vi "final_control_mk10_040325.vi"() -> ()   [LabVIEW 2023]
doc: "Simplified example program for initializing the COM port, determining the data frame of up to 26 Alicats, acquiring the data of the same number of Alicats, displaying the data of the one with the selected unit ID, and writing a setpoint to the same selected unit ID.\n\nThis is a slightly more feature rich version of the Alicat Simplified Driver Example, and contains an example of a method for interfacing with up to 26 Alicats on a single COM port by means of for loops with shift registers to handle sequential commands to each included Alicat. This also contains a method to write a setpoint to the same selected unit.\n\nIf coding for multiple Alicats on a single COM port without the use of for loops with shift registers, ensure that each Alicat command is executed sequentially. Alicat's RS-232/485 does not work if multiple devices are responding simultaneously."
uses:
  <vilib>/Platform/TimedLoop/XDataNode/timing_clust.ctl
  <vilib>/Platform/TimedLoop/XDataNode/nitl_modes.ctl
  <vilib>/Platform/TimedLoop/XDataNode/wakeup.ctl
  <vilib>/DAQmx/write.llb/DAQmx Write (Analog 1D DBL NChan 1Samp).vi
  <extravilib>/ChannelInstances/Tag-bool/Read With Abort.vi
  <extravilib>/ChannelInstances/Tag-bool/Write With Abort.vi
  <vilib>/Utility/file.llb/Write Delimited Spreadsheet (string).vi
  <extravilib>/ChannelInstances/Tag-bool/Instantiate.vi
  <vilib>/Utility/file.llb/Read Delimited Spreadsheet (DBL).vi
  <extravilib>/ChannelInstances/Tag-bool/EndpointRead.vi
  <vilib>/DAQmx/miscellaneous.llb/DAQmx Fill In Error Info.vi
  <extravilib>/ChannelInstances/Tag-bool/Endpoint.vi
  <vilib>/platform/TimedLoop/XDataNode/XDataNode.xnode
  <vilib>/express/express arith-compare/Formula/XNode/ExpressFormulaBlockNode.xnode
  <vilib>/DAQmx/read.llb/DAQmx Read (Analog DBL 1Chan 1Samp).vi
  <vilib>/Platform/TimedLoop/XDataNode/XDNodeRunTimeDep.lvlib
  <extravilib>/ChannelInstances/Tag-bool.lvlib
panel:
  in  "Tab Control":enum32{"Page 1", "Page 2"}(tab)
  in  "COM Port Settings":T1={"Baud Rate"=enum."19200", "VISA Sesssion In"="MassFlowControllers"}
  out "Range Exceeded":bool
  out "Error Present":bool
  out "Error Text":string
  out "Elapsed Time [ms]\n(all units)":dbl caption="Elapsed Time (s)"
  in  "Minimum time between \nreadings [ms] (all units)":u32
  in  "Device ID's \nto Include:":T2={"A"=TRUE, "B"=TRUE, "C"=TRUE, "D"=TRUE, "E"=TRUE, "F"=TRUE, "G"=FALSE, "H"=FALSE, "I"=FALSE, "J"=FALSE, "K"=FALSE, "L"=FALSE, "M"=FALSE, "N"=FALSE, "O"=FALSE, "P"=FALSE, "Q"=FALSE, "R"=FALSE, "S"=FALSE, "T"=FALSE, "U"=FALSE, "V"=FALSE, "W"=FALSE, "X"=FALSE, "Y"=FALSE, "Z"=FALSE}
  out "Active Device":u16(ring) items=["A", "B", "C", "D", "E", "F"]
  out "Meas. Data (for active device)":T3
  in  "Write File":path
  in  "Hold Time\n[min]":dbl=17.0 min=17.0
  out "N":i32
  in  "Read File":path
  in  "End Program":bool
  in  "Start From:":i32=1
  in  "t_read [ms]":dbl=24000.0
  out "T_SCh [C]":dbl format="%0.2f"
  out "iter start":string
  out "Iter_Duration [ms]":string
  out "C_SP [ppm]":string
  out "C_H2S [ppm]":string
  in  "Start Times":path
  out "len_SP":i32
  out "Setpoints":dbl[][](array[numeric])=[[4.2, 3.3], [69.0, 4.2]]
  out "Z":dbl[](array[numeric])
  out "ASP":dbl
  out "BSP":dbl
  out "CSP":dbl
  out "DSP":dbl
  out "ESP":dbl
  out "FSP":dbl
  out "N_read":i32
  out "Iter_#":string
  out "V_D":string
  out "V_H":string
  out "all rows":dbl[][](array[numeric])
  out "T_SCh":string
  out "Iteration Duration":i64
  out "read_cnt_true":i32
  out "iter_dur_read [ms]":i64
  out "t_diff":dbl
  out "date":string
  out "time":string
  # "Totalizer Timer"
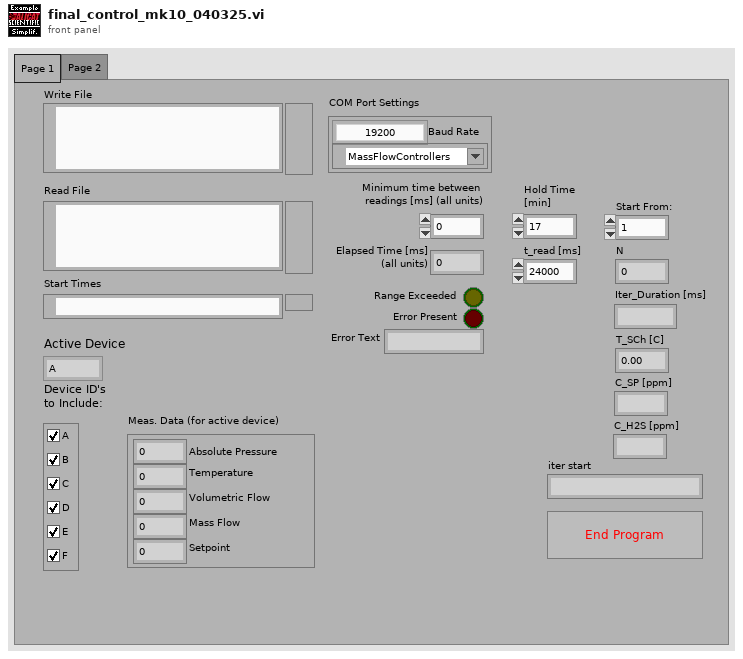
[diagram p1: front panel]
types:
  T1 = cluster{"Baud Rate":enum8{"2400", "9600", "19200", "38400", "57600", "115200", "Unknown"}, "VISA Sesssion In":refnum<visa-resource-name>}
  T2 = cluster{"A":bool, "B":bool, "C":bool, "D":bool, "E":bool, "F":bool, "G":bool, "H":bool, "I":bool, "J":bool, "K":bool, "L":bool, "M":bool, "N":bool, "O":bool, "P":bool, "Q":bool, "R":bool, "S":bool, "T":bool, "U":bool, "V":bool, "W":bool, "X":bool, "Y":bool, "Z":bool}
  T3 = cluster{"Absolute Pressure":dbl, "Gauge/Diff. Pressure":dbl, "Barometric Pressure":dbl, "Temperature":dbl, "Volumetric Flow":dbl, "Mass Flow":dbl, "Setpoint":dbl, "Valve Drive":dbl, "Totalizer":dbl, "[hr]":dbl, "[min]":dbl, "[sec]":dbl, "Totalizer Average Flow":dbl, "Totalizer Peak Flow":dbl, "Gas selected":string}
  T4 = cluster{"Unit ID":string, "Baud Rate":enum8{"2400", "9600", "19200", "38400", "57600", "115200", "Unknown"}, "VISA Sesssion In":refnum<visa-resource-name>}
  T5 = enum16{"Request Ack", "Set Setpoint", "Set Lo Limit", "Set Hi Limit", "Set Prop Band 0-99.9", "Set Integral 0-9.99", "Set Derivative 0-5.0", "Read Int Temp", "Read Ext Temp", "Read Setpoint", "Read Low Limit", "Read High Limit", "Read Prop Band", "Read Integral", "Read Derivative "}
  T6 = typedef "XDNodeRunTimeDep.lvlib/timing_clust.ctl" = cluster{"Expected End [f-1]":u64, "Actual End [f-1]":u64, "Finished Late? [f-1]":bool, "Expected End [i-1]":u64, "Actual End [i-1]":u64, "Finished Late? [i-1]":bool, "Expected Start [i]":u64, "Actual Start [i]":u64, "Expected Start [f]":u64, "Actual Start [f]":u64, "Source Name":string, "Structure Name":string, "Period":i64, "Deadline":i64, "Offset":i64, "Start":i64, "Priority":i32, "Timeout":i32, "Mode":T7, "Wakeup Reason":T8, "Error":errorcluster, "Source Type":string, "Secondary Source Type":string, "Global End Time":u64, "Global Start Time":u64, "Frame Duration":u64, "Iteration Duration":u64, "Assigned CPU":i32, "I/O Scan Engine Mode":u32}
  T7 = typedef "XDNodeRunTimeDep.lvlib/nitl_modes.ctl" = enum32{"No Change", "Process missed periods, maintain original phase", "Discard missed periods, maintain original phase", "Process missed periods, ignore original phase", "Discard missed periods, ignore original phase"}
  T8 = typedef "XDNodeRunTimeDep.lvlib/wakeup.ctl" = enum32{"Normal", "Aborted", "Asynchronous wakeup", "Timing source error", "Timed loop error", "Timeout"}
  T9 = typedef "Tag-bool.lvlib/))Channel.ctl" = refnum<queue>
  T10 = enum8{"2400", "9600", "19200", "38400", "57600", "115200", "Unknown"}
  T11 = cluster{"Absolute Pressure":bool, "Gauge/Diff. Pressure":bool, "Barometric Pressure":bool, "Temperature":bool, "Volumetric":bool, "Mass":bool, "Setpoint":bool, "Valve Drive":bool, "Totalizer":bool, "Totalizer Timer":bool, "Totalizer Average Flow":bool, "Totalizer Peak Flow":bool, "Gas Selected":bool, "Tot. Timer Format":u16}
  T12 = cluster{"Controller Full Scale":dbl, "Controller Select":u16, "Control Range":enum16{"Normal", "Inverted", "Bidirectional", "Unknown"}}
  T13 = cluster{"Controller Full Scale":dbl, "Controller Select":u16, "Control Range":enum16{"Normal", "Inverted", "Bidirectional", "Unknown"}}[]
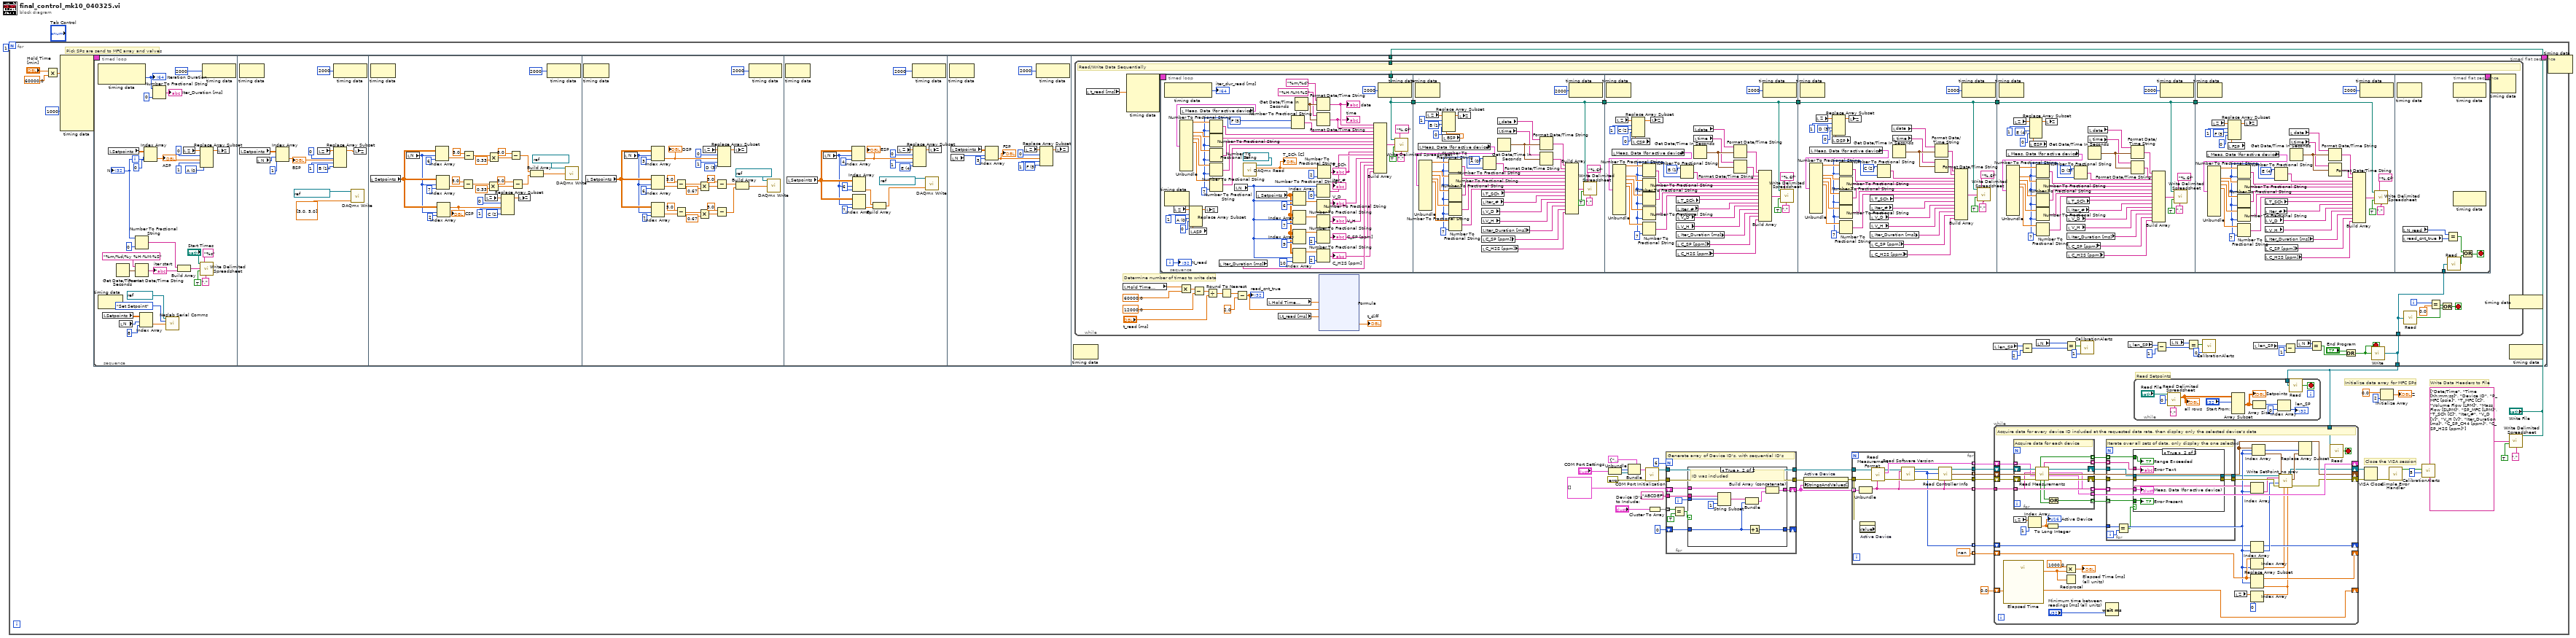
[diagram p0: block diagram]
diagram:
  n1 = for {
    N: 1 -> [_]
    # "Pick SPs are send to MFC array and valves"
    # "Write Data Headers to File"
    # "Read Setpoints"
    # "Initialize data array for MFC SPs"
    # "Close the VISA session"
    n2 = Multiply(x="Hold Time\n[min]", y=60000.0) -> (x*y=w5:dbl)
    n3 = node-c288(w5, i64 1000 ("Offset")) -> (w46:T6)  [unwired: 8 in]
    n4 = timed-loop "Write Data" {
      timing: w46 -> [_]
      timing-out: [_] -> w45
      tunnel: [w59] -> w12
      tunnel: "Write File" -> [w58]
      i -> [w73]
      stop <- w227 stop-if-true
      n5 = timed-sequence {
        timing: _ -> [_]
        timing-out: _ -> [_]
        tunnel: [w61] -> w59
        tunnel: w58 -> [w60]
        n6 = timed-flat-sequence {
          tunnel: [w222] -> w61
          tunnel: w60 -> [w223]
          frame #0 {
            w83 = u16 0 items=["A", "B", "C", "D", "E", "F"]
            n7 = node-c288() -> (w77:i64)  [unwired: 1 in, 1 out]
            "Iteration Duration" <- w77
            n8 = local read "Setpoints"() -> (w67:dbl[][])
            n9 = local read "Setpoints"() -> (w90:dbl[][])
            n10 = Get Date/Time In Seconds() -> (seconds since 1Jan1904=w78:timestamp)
            n11 = local read "N"() -> (w66:i32)
            n12 = Number To Fractional String(number=w73, precision (6)=i16 0) -> (F-format string=w71:string)  [unwired: 2 in]
            n13 = Format Date/Time String(time format string (%c)="%m/%d/%y %H:%M:%S", seconds (now)=w78) -> (date/time string=w70:string)  [unwired: 1 in]
            "iter start" <- w70
            n14 = Index Array(array=w67, index (row)=w66, index (col)=8 ("disabled index (col)")) -> (element=w64:dbl)
            n15 = Index Array(array=w90, index (row)=w73, index (col)=0 ("index (row)")) -> (element=w88:dbl)
            "ASP" <- w88
            n16 = Number To Fractional String(number=w77, precision (6)=i16 0) -> (F-format string=→"Iter_Duration [ms]":string)  [unwired: 2 in]
            n17 = call "Neslab Serial Comms.vi"("VISA resource name"=refnum<visa-resource-name> "COM1", "Command"=T5."Set Setpoint", "Set Value"=w64) -> ()  [unwired: 6 in, 7 out]
            n18 = Build Array(w71, w70) -> (w69:string[])
            n19 = local read "Z"() -> (w86:dbl[])
            n20 = Replace Array Subset(array=w86, new element #1=w88, index #1=0 ("index"), new element #2=w83, index #2=1 ("index")) -> (w87:dbl[])
            n21 = call-poly <vilib>:"Write Delimited Spreadsheet.vi"("file path (dialog if empty)"="Start Times", "format (%s)"="%s" ("format (%.3f)"), "1D data"=w69, "append to file? (new file:F)"=TRUE, "delimiter (\\t)"="," ("delimiter (\\t)")) -> ()  [unwired: 9 in, 2 out]
            n22 = node-c288(i64 2000 ("Start")) -> ()  [unwired: 1 out]
            n23 = local write "Z"(w87) -> ()
            "N" <- w73
          }
          frame #1 {
            w98 = u16 1 items=["A", "B", "C", "D", "E", "F"]
            n24 = node-c288() -> ()  [unwired: 1 in, 1 out]
            n25 = local read "Setpoints"() -> (w106:dbl[][])
            n26 = local read "N"() -> (w99:i32)
            n27 = Index Array(array=w106, index (row)=w99, index (col)=1 ("index (row)")) -> (element=w103:dbl)
            "BSP" <- w103
            n28 = local read "Z"() -> (w101:dbl[])
            n29 = Replace Array Subset(array=w101, new element #1=w103, index #1=0 ("index"), new element #2=w98, index #2=1 ("index")) -> (w102:dbl[])
            n30 = node-c288(i64 2000 ("Start")) -> ()  [unwired: 1 out]
            n31 = call-poly <vilib>:"DAQmx Write.vi"("task/channels in"=refnum<k21> "Valve_cont", "data"=dbl[] [5.0, 5.0]) -> ()  [unwired: 11 in, 3 out]
            n32 = local write "Z"(w102) -> ()
          }
          frame #2 {
            w113 = u16 2 items=["A", "B", "C", "D", "E", "F"]
            n33 = node-c288() -> ()  [unwired: 1 in, 1 out]
            n34 = local read "Setpoints"() -> (w125:dbl[][])
            n35 = local read "N"() -> (w124:i32)
            n36 = Index Array(array=w125, index (row)=w124, index (col)=6 ("disabled index (col)")) -> (element=w115:dbl)
            n37 = Index Array(array=w125, index (row)=w124, index (col)=7 ("disabled index (col)")) -> (element=w123:dbl)
            n38 = Index Array(array=w125, index (row)=w124, index (col)=2 ("index (row)")) -> (element=w137:dbl)
            "CSP" <- w137
            n39 = Subtract(x=5.0, y=w123) -> (x-y=w132:dbl)
            n40 = Subtract(x=5.0, y=w115) -> (x-y=w119:dbl)
            n41 = local read "Z"() -> (w135:dbl[])
            n42 = Multiply(x=w132, y=0.33) -> (x*y=w130:dbl)
            n43 = Multiply(x=w119, y=0.33) -> (x*y=w117:dbl)
            n44 = Replace Array Subset(array=w135, new element #1=w137, index #1=0 ("index"), new element #2=w113, index #2=1 ("index")) -> (w136:dbl[])
            n45 = Subtract(x=5.0, y=w117) -> (x-y=w114:dbl)
            n46 = Subtract(x=5.0, y=w130) -> (x-y=w127:dbl)
            n47 = local write "Z"(w136) -> ()
            n48 = Build Array(w114, w127) -> (w126:dbl[])
            n49 = node-c288(i64 2000 ("Start")) -> ()  [unwired: 1 out]
            n50 = call-poly <vilib>:"DAQmx Write.vi"("task/channels in"=refnum<k21> "Valve_cont", "data"=w126) -> ()  [unwired: 11 in, 3 out]
          }
          frame #3 {
            w164 = u16 3 items=["A", "B", "C", "D", "E", "F"]
            n51 = node-c288() -> ()  [unwired: 1 in, 1 out]
            n52 = local read "Setpoints"() -> (w153:dbl[][])
            n53 = local read "N"() -> (w152:i32)
            n54 = Index Array(array=w153, index (row)=w152, index (col)=7 ("disabled index (col)")) -> (element=w145:dbl)
            n55 = Index Array(array=w153, index (row)=w152, index (col)=3 ("index (row)")) -> (element=w168:dbl)
            "DSP" <- w168
            n56 = Index Array(array=w153, index (row)=w152, index (col)=6 ("disabled index (col)")) -> (element=w151:dbl)
            n57 = Subtract(x=5.0, y=w151) -> (x-y=w161:dbl)
            n58 = Subtract(x=5.0, y=w145) -> (x-y=w149:dbl)
            n59 = Multiply(x=w161, y=0.67) -> (x*y=w159:dbl)
            n60 = Multiply(x=w149, y=0.67) -> (x*y=w147:dbl)
            n61 = local read "Z"() -> (w166:dbl[])
            n62 = Subtract(x=5.0, y=w159) -> (x-y=w155:dbl)
            n63 = Subtract(x=5.0, y=w147) -> (x-y=w144:dbl)
            n64 = Replace Array Subset(array=w166, new element #1=w168, index #1=0 ("index"), new element #2=w164, index #2=1 ("index")) -> (w167:dbl[])
            n65 = local write "Z"(w167) -> ()
            n66 = Build Array(w155, w144) -> (w154:dbl[])
            n67 = node-c288(i64 2000 ("Start")) -> ()  [unwired: 1 out]
            n68 = call-poly <vilib>:"DAQmx Write.vi"("task/channels in"=refnum<k21> "Valve_cont", "data"=w154) -> ()  [unwired: 11 in, 3 out]
          }
          frame #4 {
            w185 = u16 4 items=["A", "B", "C", "D", "E", "F"]
            n69 = node-c288() -> ()  [unwired: 1 in, 1 out]
            n70 = local read "Setpoints"() -> (w180:dbl[][])
            n71 = local read "N"() -> (w179:i32)
            n72 = Index Array(array=w180, index (row)=w179, index (col)=4 ("index (row)")) -> (element=w189:dbl)
            "ESP" <- w189
            n73 = Index Array(array=w180, index (row)=w179, index (col)=6 ("disabled index (col)")) -> (element=w182:dbl)
            n74 = Index Array(array=w180, index (row)=w179, index (col)=7 ("disabled index (col)")) -> (element=w181:dbl)
            n75 = Build Array(w182, w181) -> (w178:dbl[])
            n76 = local read "Z"() -> (w187:dbl[])
            n77 = node-c288(i64 2000 ("Start")) -> ()  [unwired: 1 out]
            n78 = Replace Array Subset(array=w187, new element #1=w189, index #1=0 ("index"), new element #2=w185, index #2=1 ("index")) -> (w188:dbl[])
            n79 = call-poly <vilib>:"DAQmx Write.vi"("task/channels in"=refnum<k21> "Valve_cont", "data"=w178) -> ()  [unwired: 11 in, 3 out]
            n80 = local write "Z"(w188) -> ()
          }
          frame #5 {
            w199 = u16 5 items=["A", "B", "C", "D", "E", "F"]
            n81 = node-c288() -> ()  [unwired: 1 in, 1 out]
            n82 = local read "Setpoints"() -> (w202:dbl[][])
            n83 = local read "N"() -> (w197:i32)
            n84 = Index Array(array=w202, index (row)=w197, index (col)=5 ("index (row)")) -> (element=w198:dbl)
            "FSP" <- w198
            n85 = local read "Z"() -> (w201:dbl[])
            n86 = node-c288(i64 2000 ("Start")) -> ()  [unwired: 1 out]
            n87 = Replace Array Subset(array=w201, new element #1=w198, index #1=0 ("index"), new element #2=w199, index #2=1 ("index")) -> (w200:dbl[])
            n88 = local write "Z"(w200) -> ()
          }
          frame #6 {
            n89 = node-c288() -> ()  [unwired: 1 in, 1 out]
            n90 = local read "len_SP"() -> (w213:i32)
            n91 = Subtract(x=w213, y=2) -> (x-y=w215:i32)
            n92 = local read "N"() -> (w214:i32)
            n93 = Equal?(x=w214, y=w215) -> (x = y?=w211:bool)
            n94 = call "CalibrationAlerts.vi"("Alert Type (0)"=1, "Trigger"=w211) -> ()  [unwired: 10 in]
            n95 = local read "len_SP"() -> (w218:i32)
            n96 = Subtract(x=w218, y=1) -> (x-y=w217:i32)
            n97 = local read "N"() -> (w221:i32)
            n98 = Equal?(x=w221, y=w217) -> (x = y?=w210:bool)
            n99 = call "CalibrationAlerts.vi"("Alert Type (0)"=0, "Trigger"=w210) -> ()  [unwired: 10 in]
            n100 = local read "len_SP"() -> (w226:i32)
            n101 = Subtract(x=w226, y=1) -> (x-y=w229:i32)
            n102 = local read "N"() -> (w225:i32)
            n103 = Equal?(x=w225, y=w229) -> (x = y?=w228:bool)
            n104 = Or(x="End Program", y=w228) -> (x .or. y?=w227:bool)
            n105 = call <extravilib>:"Write.vi"("element"=w227) -> ("channel"=w222:T9)  [unwired: 1 out]
            n106 = while {
              tunnel: w223 -> [w251]
              tunnel: w222 -> [w241]
              i -> [w240]
              stop <- w247 stop-if-true
              # "Determine number of times to write data"
              # "Read/Write Data Sequentially"
              n107 = local read "t_read [ms]"() -> (w231:dbl)
              n108 = local read "Hold Time\n[min]"() -> (w245:dbl)
              n109 = node-c288(w231) -> (w253:T6)  [unwired: 3 in]
              n110 = timed-loop {
                timing: w253 -> [_]
                timing-out: [_] -> w252
                tunnel: w251 -> [w266]
                tunnel: w241 -> [w267]
                i -> [w330]
                stop <- w549 stop-if-true
                n111 = timed-sequence {
                  timing: _ -> [_]
                  timing-out: _ -> [_]
                  tunnel: w267 -> [w269]
                  tunnel: w266 -> [w268]
                  n112 = timed-flat-sequence {
                    tunnel: [w296] -> w274
                    tunnel: w268 -> [w296]
                    tunnel: w274 -> [w361]
                    tunnel: [w361] -> w273
                    tunnel: w273 -> [w396]
                    tunnel: [w396] -> w272
                    tunnel: w272 -> [w434]
                    tunnel: [w434] -> w271
                    tunnel: w271 -> [w466]
                    tunnel: [w466] -> w270
                    tunnel: w270 -> [w518]
                    tunnel: w269 -> [w548]
                    frame #0 {
                      w311 = u16 5 items=["A", "B", "C", "D", "E", "F"]
                      w314 = u16 0 items=["A", "B", "C", "D", "E", "F"]
                      w307 = i16 7 ("precision (6)")
                      n113 = node-c288() -> (→"iter_dur_read [ms]":i64)  [unwired: 1 in]
                      n114 = local read "Z"() -> (w300:dbl[])
                      n115 = local read "Meas. Data (for active device)"() -> (w297:T3)
                      n116 = Unbundle(w297) -> ("Absolute Pressure"=w320:dbl, "Temperature"=w310:dbl, "Volumetric Flow"=w316:dbl, "Mass Flow"=w309:dbl, "Setpoint"=w308:dbl)  [unwired: 10 out]
                      n117 = local read "ASP"() -> (w298:dbl)
                      n118 = Replace Array Subset(array=w300, new element #1=w314, index #1=1 ("index"), new element #2=w298, index #2=0 ("index")) -> (w299:dbl[])
                      n119 = local write "Z"(w299) -> ()
                      n120 = Number To Fractional String(number=w320, precision (6)=w307) -> (F-format string=w305:string)  [unwired: 2 in]
                      n121 = Number To Fractional String(number=w310, precision (6)=w307) -> (F-format string=w303:string)  [unwired: 2 in]
                      n122 = Number To Fractional String(number=w316, precision (6)=w307) -> (F-format string=w304:string)  [unwired: 2 in]
                      n123 = Number To Fractional String(number=w309, precision (6)=w307) -> (F-format string=w302:string)  [unwired: 2 in]
                      n124 = Number To Fractional String(number=w308, precision (6)=w307) -> (F-format string=w301:string)  [unwired: 2 in]
                      n125 = local read "Iter_Duration [ms]"() -> (w295:string)
                      n126 = local read "N"() -> (w277:i32)
                      n127 = call-poly <vilib>:"DAQmx Read.vi"("task/channels in"=refnum<k21> "T_SCh") -> ("data"=w323:dbl)  [unwired: 12 in, 2 out]
                      "T_SCh [C]" <- w323
                      n128 = local read "Setpoints"() -> (w276:dbl[][])
                      n129 = Number To Fractional String(number=w311, precision (6)=w307) -> (F-format string=w306:string)  [unwired: 2 in]
                      n130 = Index Array(array=w276, index (row)=w277, index (col)=6 ("disabled index (col)")) -> (element=w327:dbl)
                      n131 = Index Array(array=w276, index (row)=w277, index (col)=7 ("disabled index (col)")) -> (element=w326:dbl)
                      n132 = Index Array(array=w276, index (row)=w277, index (col)=9 ("disabled index (col)")) -> (element=w283:dbl)
                      n133 = Index Array(array=w276, index (row)=w277, index (col)=10 ("disabled index (col)")) -> (element=w279:dbl)
                      n134 = Get Date/Time In Seconds() -> (seconds since 1Jan1904=w289:timestamp)
                      n135 = Format Date/Time String(time format string (%c)="%m/%d", seconds (now)=w289) -> (date/time string=w291:string)  [unwired: 1 in]
                      "date" <- w291
                      n136 = Format Date/Time String(time format string (%c)="%H:%M:%S", seconds (now)=w289) -> (date/time string=w290:string)  [unwired: 1 in]
                      "time" <- w290
                      n137 = Number To Fractional String(number=w277, precision (6)=i16 0) -> (F-format string=w292:string)  [unwired: 2 in]
                      "Iter_#" <- w292
                      n138 = Number To Fractional String(number=w327) -> (F-format string=w293:string)  [unwired: 3 in]
                      "V_D" <- w293
                      n139 = Number To Fractional String(number=w326) -> (F-format string=w294:string)  [unwired: 3 in]
                      "V_H" <- w294
                      n140 = Number To Fractional String(number=w283, precision (6)=i16 2) -> (F-format string=w281:string)  [unwired: 2 in]
                      "C_SP [ppm]" <- w281
                      n141 = Number To Fractional String(number=w279, precision (6)=i16 2) -> (F-format string=w275:string)  [unwired: 2 in]
                      "C_H2S [ppm]" <- w275
                      n142 = Number To Fractional String(number=w323, precision (6)=i16 2) -> (F-format string=w286:string)  [unwired: 2 in]
                      "T_SCh" <- w286
                      n143 = Build Array(w291, w290, w306, w305, w303, w304, w302, w301, w286, w292, w293, w294, w295, w281, w275) -> (w317:string[])
                      n144 = node-c288(i64 2000 ("Start")) -> ()  [unwired: 1 out]
                      n145 = call-poly <vilib>:"Write Delimited Spreadsheet.vi"("file path (dialog if empty)"=w296, "format (%s)"="%.6f" ("format (%.3f)"), "1D data"=w317, "append to file? (new file:F)"=TRUE, "delimiter (\\t)"="," ("delimiter (\\t)")) -> ()  [unwired: 9 in, 2 out]
                      "N_read" <- w330
                    }
                    frame #1 {
                      w358 = u16 0 items=["A", "B", "C", "D", "E", "F"]
                      w367 = u16 1 items=["A", "B", "C", "D", "E", "F"]
                      w354 = i16 7 ("precision (6)")
                      n146 = node-c288() -> ()  [unwired: 1 in, 1 out]
                      n147 = local read "Meas. Data (for active device)"() -> (w365:T3)
                      n148 = Unbundle(w365) -> ("Absolute Pressure"=w373:dbl, "Temperature"=w357:dbl, "Volumetric Flow"=w369:dbl, "Mass Flow"=w356:dbl, "Setpoint"=w355:dbl)  [unwired: 10 out]
                      n149 = local read "Z"() -> (w364:dbl[])
                      n150 = local read "BSP"() -> (w359:dbl)
                      n151 = Replace Array Subset(array=w364, new element #1=w367, index #1=1 ("index"), new element #2=w359, index #2=0 ("index")) -> (w363:dbl[])
                      n152 = Number To Fractional String(number=w373, precision (6)=w354) -> (F-format string=w352:string)  [unwired: 2 in]
                      n153 = Number To Fractional String(number=w357, precision (6)=w354) -> (F-format string=w350:string)  [unwired: 2 in]
                      n154 = Number To Fractional String(number=w369, precision (6)=w354) -> (F-format string=w351:string)  [unwired: 2 in]
                      n155 = Number To Fractional String(number=w356, precision (6)=w354) -> (F-format string=w349:string)  [unwired: 2 in]
                      n156 = Number To Fractional String(number=w355, precision (6)=w354) -> (F-format string=w348:string)  [unwired: 2 in]
                      n157 = local write "Z"(w363) -> ()
                      n158 = local read "T_SCh"() -> (w347:string)
                      n159 = local read "Iter_#"() -> (w346:string)
                      n160 = local read "V_D"() -> (w345:string)
                      n161 = local read "V_H"() -> (w344:string)
                      n162 = local read "Iter_Duration [ms]"() -> (w343:string)
                      n163 = local read "C_SP [ppm]"() -> (w337:string)
                      n164 = local read "C_H2S [ppm]"() -> (w336:string)
                      n165 = Number To Fractional String(number=w358, precision (6)=w354) -> (F-format string=w353:string)  [unwired: 2 in]
                      n166 = local read "date"() -> (w338:string)
                      n167 = local read "time"() -> (w339:string)
                      n168 = Get Date/Time In Seconds() -> (seconds since 1Jan1904=w340:timestamp)
                      n169 = Format Date/Time String(time format string (%c)=w338, seconds (now)=w340) -> (date/time string=w342:string)  [unwired: 1 in]
                      n170 = Format Date/Time String(time format string (%c)=w339, seconds (now)=w340) -> (date/time string=w341:string)  [unwired: 1 in]
                      n171 = Build Array(w342, w341, w353, w352, w350, w351, w349, w348, w347, w346, w345, w344, w343, w337, w336) -> (w370:string[])
                      n172 = node-c288(i64 2000 ("Start")) -> ()  [unwired: 1 out]
                      n173 = call-poly <vilib>:"Write Delimited Spreadsheet.vi"("file path (dialog if empty)"=w361, "format (%s)"="%.6f" ("format (%.3f)"), "1D data"=w370, "append to file? (new file:F)"=TRUE, "delimiter (\\t)"="," ("delimiter (\\t)")) -> ()  [unwired: 9 in, 2 out]
                    }
                    frame #2 {
                      w402 = u16 1 items=["A", "B", "C", "D", "E", "F"]
                      w401 = i16 7 ("precision (6)")
                      w414 = u16 2 items=["A", "B", "C", "D", "E", "F"]
                      n174 = node-c288() -> ()  [unwired: 1 in, 1 out]
                      n175 = local read "Meas. Data (for active device)"() -> (w403:T3)
                      n176 = Unbundle(w403) -> ("Absolute Pressure"=w408:dbl, "Temperature"=w406:dbl, "Volumetric Flow"=w407:dbl, "Mass Flow"=w405:dbl, "Setpoint"=w404:dbl)  [unwired: 10 out]
                      n177 = local read "Z"() -> (w413:dbl[])
                      n178 = local read "CSP"() -> (w409:dbl)
                      n179 = Replace Array Subset(array=w413, new element #1=w414, index #1=1 ("index"), new element #2=w409, index #2=0 ("index")) -> (w412:dbl[])
                      n180 = Number To Fractional String(number=w408, precision (6)=w401) -> (F-format string=w389:string)  [unwired: 2 in]
                      n181 = Number To Fractional String(number=w406, precision (6)=w401) -> (F-format string=w388:string)  [unwired: 2 in]
                      n182 = Number To Fractional String(number=w407, precision (6)=w401) -> (F-format string=w387:string)  [unwired: 2 in]
                      n183 = Number To Fractional String(number=w405, precision (6)=w401) -> (F-format string=w386:string)  [unwired: 2 in]
                      n184 = Number To Fractional String(number=w404, precision (6)=w401) -> (F-format string=w385:string)  [unwired: 2 in]
                      n185 = local write "Z"(w412) -> ()
                      n186 = local read "T_SCh"() -> (w395:string)
                      n187 = local read "Iter_#"() -> (w394:string)
                      n188 = local read "V_D"() -> (w393:string)
                      n189 = local read "V_H"() -> (w392:string)
                      n190 = local read "Iter_Duration [ms]"() -> (w391:string)
                      n191 = local read "C_SP [ppm]"() -> (w379:string)
                      n192 = local read "C_H2S [ppm]"() -> (w378:string)
                      n193 = Number To Fractional String(number=w402, precision (6)=w401) -> (F-format string=w390:string)  [unwired: 2 in]
                      n194 = local read "date"() -> (w380:string)
                      n195 = local read "time"() -> (w381:string)
                      n196 = Get Date/Time In Seconds() -> (seconds since 1Jan1904=w382:timestamp)
                      n197 = Format Date/Time String(time format string (%c)=w380, seconds (now)=w382) -> (date/time string=w384:string)  [unwired: 1 in]
                      n198 = Format Date/Time String(time format string (%c)=w381, seconds (now)=w382) -> (date/time string=w383:string)  [unwired: 1 in]
                      n199 = Build Array(w384, w383, w390, w389, w388, w387, w386, w385, w395, w394, w393, w392, w391, w379, w378) -> (w397:string[])
                      n200 = node-c288(i64 2000 ("Start")) -> ()  [unwired: 1 out]
                      n201 = call-poly <vilib>:"Write Delimited Spreadsheet.vi"("file path (dialog if empty)"=w396, "format (%s)"="%.6f" ("format (%.3f)"), "1D data"=w397, "append to file? (new file:F)"=TRUE, "delimiter (\\t)"="," ("delimiter (\\t)")) -> ()  [unwired: 9 in, 2 out]
                    }
                    frame #3 {
                      w428 = u16 3 items=["A", "B", "C", "D", "E", "F"]
                      w451 = u16 2 items=["A", "B", "C", "D", "E", "F"]
                      w450 = i16 7 ("precision (6)")
                      n202 = node-c288() -> ()  [unwired: 1 in, 1 out]
                      n203 = local read "Meas. Data (for active device)"() -> (w433:T3)
                      n204 = Unbundle(w433) -> ("Absolute Pressure"=w456:dbl, "Temperature"=w454:dbl, "Volumetric Flow"=w455:dbl, "Mass Flow"=w453:dbl, "Setpoint"=w452:dbl)  [unwired: 10 out]
                      n205 = local read "Z"() -> (w431:dbl[])
                      n206 = local read "DSP"() -> (w432:dbl)
                      n207 = Replace Array Subset(array=w431, new element #1=w428, index #1=1 ("index"), new element #2=w432, index #2=0 ("index")) -> (w430:dbl[])
                      n208 = Number To Fractional String(number=w456, precision (6)=w450) -> (F-format string=w444:string)  [unwired: 2 in]
                      n209 = Number To Fractional String(number=w454, precision (6)=w450) -> (F-format string=w443:string)  [unwired: 2 in]
                      n210 = Number To Fractional String(number=w455, precision (6)=w450) -> (F-format string=w442:string)  [unwired: 2 in]
                      n211 = Number To Fractional String(number=w453, precision (6)=w450) -> (F-format string=w441:string)  [unwired: 2 in]
                      n212 = Number To Fractional String(number=w452, precision (6)=w450) -> (F-format string=w440:string)  [unwired: 2 in]
                      n213 = local write "Z"(w430) -> ()
                      n214 = local read "T_SCh"() -> (w435:string)
                      n215 = local read "Iter_#"() -> (w436:string)
                      n216 = local read "V_D"() -> (w437:string)
                      n217 = local read "V_H"() -> (w438:string)
                      n218 = local read "Iter_Duration [ms]"() -> (w439:string)
                      n219 = local read "C_SP [ppm]"() -> (w421:string)
                      n220 = local read "C_H2S [ppm]"() -> (w420:string)
                      n221 = Number To Fractional String(number=w451, precision (6)=w450) -> (F-format string=w445:string)  [unwired: 2 in]
                      n222 = local read "date"() -> (w422:string)
                      n223 = local read "time"() -> (w423:string)
                      n224 = Get Date/Time In Seconds() -> (seconds since 1Jan1904=w424:timestamp)
                      n225 = Format Date/Time String(time format string (%c)=w422, seconds (now)=w424) -> (date/time string=w426:string)  [unwired: 1 in]
                      n226 = Format Date/Time String(time format string (%c)=w423, seconds (now)=w424) -> (date/time string=w425:string)  [unwired: 1 in]
                      n227 = Build Array(w426, w425, w445, w444, w443, w442, w441, w440, w435, w436, w437, w438, w439, w421, w420) -> (w446:string[])
                      n228 = node-c288(i64 2000 ("Start")) -> ()  [unwired: 1 out]
                      n229 = call-poly <vilib>:"Write Delimited Spreadsheet.vi"("file path (dialog if empty)"=w434, "format (%s)"="%.6f" ("format (%.3f)"), "1D data"=w446, "append to file? (new file:F)"=TRUE, "delimiter (\\t)"="," ("delimiter (\\t)")) -> ()  [unwired: 9 in, 2 out]
                    }
                    frame #4 {
                      w474 = u16 4 items=["A", "B", "C", "D", "E", "F"]
                      w493 = u16 3 items=["A", "B", "C", "D", "E", "F"]
                      w492 = i16 7 ("precision (6)")
                      n230 = node-c288() -> ()  [unwired: 1 in, 1 out]
                      n231 = local read "Meas. Data (for active device)"() -> (w476:T3)
                      n232 = Unbundle(w476) -> ("Absolute Pressure"=w498:dbl, "Temperature"=w496:dbl, "Volumetric Flow"=w497:dbl, "Mass Flow"=w495:dbl, "Setpoint"=w494:dbl)  [unwired: 10 out]
                      n233 = local read "Z"() -> (w471:dbl[])
                      n234 = local read "ESP"() -> (w472:dbl)
                      n235 = Replace Array Subset(array=w471, new element #1=w474, index #1=1 ("index"), new element #2=w472, index #2=0 ("index")) -> (w470:dbl[])
                      n236 = Number To Fractional String(number=w498, precision (6)=w492) -> (F-format string=w486:string)  [unwired: 2 in]
                      n237 = Number To Fractional String(number=w496, precision (6)=w492) -> (F-format string=w485:string)  [unwired: 2 in]
                      n238 = Number To Fractional String(number=w497, precision (6)=w492) -> (F-format string=w484:string)  [unwired: 2 in]
                      n239 = Number To Fractional String(number=w495, precision (6)=w492) -> (F-format string=w483:string)  [unwired: 2 in]
                      n240 = Number To Fractional String(number=w494, precision (6)=w492) -> (F-format string=w482:string)  [unwired: 2 in]
                      n241 = local write "Z"(w470) -> ()
                      n242 = local read "T_SCh"() -> (w481:string)
                      n243 = local read "Iter_#"() -> (w477:string)
                      n244 = local read "V_D"() -> (w478:string)
                      n245 = local read "V_H"() -> (w479:string)
                      n246 = local read "Iter_Duration [ms]"() -> (w480:string)
                      n247 = local read "C_SP [ppm]"() -> (w463:string)
                      n248 = local read "C_H2S [ppm]"() -> (w462:string)
                      n249 = Number To Fractional String(number=w493, precision (6)=w492) -> (F-format string=w487:string)  [unwired: 2 in]
                      n250 = local read "date"() -> (w464:string)
                      n251 = local read "time"() -> (w465:string)
                      n252 = Get Date/Time In Seconds() -> (seconds since 1Jan1904=w467:timestamp)
                      n253 = Format Date/Time String(time format string (%c)=w464, seconds (now)=w467) -> (date/time string=w469:string)  [unwired: 1 in]
                      n254 = Format Date/Time String(time format string (%c)=w465, seconds (now)=w467) -> (date/time string=w468:string)  [unwired: 1 in]
                      n255 = Build Array(w469, w468, w487, w486, w485, w484, w483, w482, w481, w477, w478, w479, w480, w463, w462) -> (w488:string[])
                      n256 = node-c288(i64 2000 ("Start")) -> ()  [unwired: 1 out]
                      n257 = call-poly <vilib>:"Write Delimited Spreadsheet.vi"("file path (dialog if empty)"=w466, "format (%s)"="%.6f" ("format (%.3f)"), "1D data"=w488, "append to file? (new file:F)"=TRUE, "delimiter (\\t)"="," ("delimiter (\\t)")) -> ()  [unwired: 9 in, 2 out]
                    }
                    frame #5 {
                      w516 = u16 5 items=["A", "B", "C", "D", "E", "F"]
                      w536 = u16 4 items=["A", "B", "C", "D", "E", "F"]
                      w535 = i16 7 ("precision (6)")
                      n258 = node-c288() -> ()  [unwired: 1 in, 1 out]
                      n259 = local read "Meas. Data (for active device)"() -> (w519:T3)
                      n260 = Unbundle(w519) -> ("Absolute Pressure"=w541:dbl, "Temperature"=w539:dbl, "Volumetric Flow"=w540:dbl, "Mass Flow"=w538:dbl, "Setpoint"=w537:dbl)  [unwired: 10 out]
                      n261 = local read "Z"() -> (w512:dbl[])
                      n262 = local read "FSP"() -> (w514:dbl)
                      n263 = Replace Array Subset(array=w512, new element #1=w516, index #1=1 ("index"), new element #2=w514, index #2=0 ("index")) -> (w513:dbl[])
                      n264 = Number To Fractional String(number=w541, precision (6)=w535) -> (F-format string=w529:string)  [unwired: 2 in]
                      n265 = Number To Fractional String(number=w539, precision (6)=w535) -> (F-format string=w528:string)  [unwired: 2 in]
                      n266 = Number To Fractional String(number=w540, precision (6)=w535) -> (F-format string=w527:string)  [unwired: 2 in]
                      n267 = Number To Fractional String(number=w538, precision (6)=w535) -> (F-format string=w526:string)  [unwired: 2 in]
                      n268 = Number To Fractional String(number=w537, precision (6)=w535) -> (F-format string=w525:string)  [unwired: 2 in]
                      n269 = local write "Z"(w513) -> ()
                      n270 = local read "T_SCh"() -> (w520:string)
                      n271 = local read "Iter_#"() -> (w521:string)
                      n272 = local read "V_D"() -> (w522:string)
                      n273 = local read "V_H"() -> (w523:string)
                      n274 = local read "Iter_Duration [ms]"() -> (w524:string)
                      n275 = local read "C_SP [ppm]"() -> (w506:string)
                      n276 = local read "C_H2S [ppm]"() -> (w505:string)
                      n277 = Number To Fractional String(number=w536, precision (6)=w535) -> (F-format string=w530:string)  [unwired: 2 in]
                      n278 = local read "date"() -> (w507:string)
                      n279 = local read "time"() -> (w508:string)
                      n280 = Get Date/Time In Seconds() -> (seconds since 1Jan1904=w509:timestamp)
                      n281 = Format Date/Time String(time format string (%c)=w507, seconds (now)=w509) -> (date/time string=w511:string)  [unwired: 1 in]
                      n282 = Format Date/Time String(time format string (%c)=w508, seconds (now)=w509) -> (date/time string=w510:string)  [unwired: 1 in]
                      n283 = Build Array(w511, w510, w530, w529, w528, w527, w526, w525, w520, w521, w522, w523, w524, w506, w505) -> (w531:string[])
                      n284 = node-c288(i64 2000 ("Start")) -> ()  [unwired: 1 out]
                      n285 = call-poly <vilib>:"Write Delimited Spreadsheet.vi"("file path (dialog if empty)"=w518, "format (%s)"="%.6f" ("format (%.3f)"), "1D data"=w531, "append to file? (new file:F)"=TRUE, "delimiter (\\t)"="," ("delimiter (\\t)")) -> ()  [unwired: 9 in, 2 out]
                    }
                    frame #6 {
                      n286 = node-c288() -> ()  [unwired: 1 in, 1 out]
                      n287 = local read "N_read"() -> (w546:i32)
                      n288 = local read "read_cnt_true"() -> (w547:i32)
                      n289 = Equal?(x=w546, y=w547) -> (x = y?=w551:bool)
                      n290 = call <extravilib>:"Read.vi"("channel"=w548) -> ("element"=w550:bool)  [unwired: 1 in, 1 out]
                      n291 = node-c288() -> ()  [unwired: 1 in, 1 out]
                      n292 = Or(x=w551, y=w550) -> (x .or. y?=w549:bool)
                    }
                  }
                }
                n293 = node-c288() -> ()  [unwired: 1 in, 1 out]
                n294 = node-c288() -> ()  [unwired: 1 in, 1 out]
              }
              n295 = Multiply(x=w245, y=60000.0) -> (x*y=w244:dbl)
              n296 = Subtract(x=w244, y=12000.0) -> (x-y=w242:dbl)
              n297 = Divide(x=w242, y="t_read [ms]") -> (x/y=w238:dbl)
              n298 = Round To Nearest(number=w238) -> (nearest integer value=w237:dbl)
              n299 = Subtract(x=w237, y=2.0) -> (x-y=w232:dbl)
              "read_cnt_true" <- w232
              n300 = local read "Hold Time\n[min]"() -> (w234:dbl)
              n301 = local read "t_read [ms]"() -> (w233:dbl)
              n302 = xnode "Formula"("X1"=w234, "X2"=w232, "X3"=w233) -> ("Result"=→"t_diff":dbl)  [unwired: 1 in, 1 out]
              n303 = call <extravilib>:"Read.vi"("channel"=w241) -> ("element"=w248:bool)  [unwired: 1 in, 1 out]
              n304 = Equal?(x=w240, y=0.0) -> (x = y?=w249:bool)
              n305 = Or(x=w249, y=w248) -> (x .or. y?=w247:bool)
              n306 = node-c288(w252) -> ()  [unwired: 1 out]
            }
            n307 = node-c288() -> ()  [unwired: 1 in, 1 out]
          }
        }
      }
      n308 = node-c288() -> ()  [unwired: 1 in, 1 out]
      n309 = node-c288() -> ()  [unwired: 1 in, 1 out]
    }
    n310 = Unbundle("COM Port Settings") -> ("Baud Rate"=w37:T10, "VISA Sesssion In"=w36:refnum<visa-resource-name>)
    n311 = Bundle(cluster=T4 {"Unit ID"="A", "Baud Rate"=enum."19200", "VISA Sesssion In"="COM1"} ("Communication Settings"), "Baud Rate"=w37, "VISA Sesssion In"=w36) -> (w35:T4)  [unwired: 1 in]
    n312 = call "COM Port Initialization.vi"("error in (no error)"=errorcluster {"status"=FALSE, "code"=0, "source"=""}, "Communication Settings"=w35) -> ("error out"=w28:errorcluster, "VISA Session Out"=w27:refnum<visa-resource-name>)  [unwired: 8 in]
    n313 = Cluster To Array(cluster="Device ID's \nto Include:") -> (array=w31:bool[])
    n314 = for {
      N: 6 -> [_]
      tunnel: "ABCDEF" -> [w593]
      tunnel: w31 -> [w586] mode=indexing
      shift-right: [w585] -> _
      shift-left: u16 0 ("length (rest)") -> [w591]
      shift-right: [w590] -> w25
      shift-left: cluster{string, u16}[] [] -> [w589]
      tunnel: w28 -> [w584]
      tunnel: w27 -> [w583]
      tunnel: [w584] -> w18
      tunnel: [w583] -> w26
      i -> [w592]
      # "Generate array of Device ID's, with sequential ID's"
      n315 = Equal?(x=w586, y=TRUE) -> (x = y?=w588:bool)
      n316 = case shown="True" w588 {
        tunnel: w593 -> [_ w604]
        tunnel: w592 -> [_ w603]
        tunnel: w591 -> [w594 w596]
        tunnel: [w595 w599] -> w590
        tunnel: w589 -> [w595 w597]
        tunnel: [w594 w600] -> w585
        frame False {
          # "ID was not included"
        }
        frame True {
          # "ID was included"
          n317 = String Subset(string=w604, offset (0)=w603, length (rest)=1 ("length (rest)")) -> (substring=w601:string)
          n318 = Bundle(w601, "length (rest)"=w596) -> (w598:cluster{string, "length (rest)":u16})  [unwired: 1 in]
          n319 = Increment(x=w596) -> (x+1=w600:u16)
          n320 = Build Array (concatenate)(w597, w598) -> (w599:cluster{string, "length (rest)":u16}[])
        }
      }
    }
    n321 = property on="Active Device" class="Ring (strict)"(error in=w18, "StringsAndValues[]"=w25) -> (error out=w17:errorcluster)  [unwired: 1 in, 1 out]
    n322 = for {
      tunnel: w26 -> [w581]
      tunnel: [w578] -> w22
      tunnel: w17 -> [w582]
      tunnel: [w577] -> w21
      tunnel: w25 -> [w579] mode=indexing
      tunnel: [w580] -> w24 mode=indexing
      tunnel: [w570] -> w23 mode=indexing
      tunnel: [w576] -> w20 mode=indexing
      tunnel: [nan ("Setpoint")] -> w19 mode=indexing
      tunnel: [w569] -> w16 mode=indexing
      # "Get measurement formats, unit ID's and the controller info"
      n323 = Unbundle(w579) -> (w570:string)  [unwired: 1 out]
      n324 = property on="Active Device" class="Ring (strict)" props=["Value"]() -> ()  [unwired: 2 in, 3 out]
      n325 = call "Read Measurement Format.vi"("Unit ID (A)"=w570, "error in"=w582, "VISA Session In"=w581) -> ("error out"=w573:errorcluster, "Data Frame Format"=w580:T11, "VISA Session Out"=w574:refnum<visa-resource-name>)  [unwired: 6 in]
      n326 = call "Read Software Version.vi"("Unit ID (A)"=w570, "error in"=w573, "VISA Session In"=w574) -> ("error out"=w572:errorcluster, "Software Version"=w569:u8, "VISA Session Out"=w571:refnum<visa-resource-name>)  [unwired: 6 in]
      n327 = call "Read Controller Info.vi"("Unit ID (A)"=w570, "error in"=w572, "Software Version"=w569, "VISA Session In"=w571) -> ("error out"=w577:errorcluster, "Controller Info out"=w576:T12, "VISA Session Out"=w578:refnum<visa-resource-name>)  [unwired: 4 in, 1 out]
    }
    n328 = while {
      shift-right: [w641] -> _
      shift-left: 0.0 ("Set Start Time (s)") -> [w644]
      shift-right: [w627] -> w40
      shift-left: w21 -> [w643]
      shift-right: [w608] -> w41
      shift-left: w22 -> [w642]
      tunnel: w23 -> [w606]
      shift-right: [w629] -> _
      shift-left: w24 -> [w636]
      shift-right: [w626] -> _
      shift-left: w20 -> [w624]
      shift-right: [w622] -> _
      shift-left: w19 -> [w621]
      shift-right: [w617] -> _
      shift-left: w16 -> [w617]
      tunnel: w12 -> [w615]
      stop <- w616 stop-if-true
      # "Acquire data for every device ID included at the requested data rate, then display only the selected device's data"
      n329 = call "Elapsed Time"("Set Start Time (s)"=w644) -> ("Get Start Time (s)"=w641:dbl, "Elapsed Time (s)"=w638:dbl)  [unwired: 11 in, 6 out]
      n330 = for {
        shift-right: [w673] -> w635
        shift-left: w643 -> [w676]
        shift-right: [w674] -> w634
        shift-left: w642 -> [w675]
        tunnel: w636 -> [w670] mode=indexing
        tunnel: w606 -> [w669] mode=indexing
        tunnel: [w668] -> w633 mode=indexing
        tunnel: [w667] -> w632 mode=indexing
        tunnel: [w666] -> w631 mode=indexing
        tunnel: [w665] -> w630 mode=indexing
        tunnel: [w664] -> w629 mode=indexing
        # "Acquire data for each device"
        n331 = call "Read Measurements.vi"("error in"=w676, "Data Frame Format In"=w670, "Unit ID (A)"=w669, "VISA Session In"=w675) -> ("error out"=w673:errorcluster, "Data Frame Format Out"=w664:T11, "Data Cluster"=w667:T3, "VISA Session Out"=w674:refnum<visa-resource-name>, "Unknown Dataframe Info"=w672:bool, "Error/Overrange/Unknown String"=w666:string, "Error Present"=w671:bool, "Range Exceeded"=w665:bool)
        n332 = Or(x=w672, y=w671) -> (x .or. y?=w668:bool)
      }
      n333 = local read "Z"() -> (w612:dbl[])
      n334 = Index Array(array=w612, index=1 ("index (row)")) -> (element=w610:dbl)
      "Active Device" <- w610
      n335 = To Long Integer(number=w610) -> (32bit integer=w619:i32)
      n336 = Multiply(x=1000.0 ("y"), y=w638) -> (x*y=→"Elapsed Time [ms]\n(all units)":dbl)
      n337 = Reciprocal(x=w638) -> ()  [unwired: 1 out]
      n338 = Wait (ms)(milliseconds to wait="Minimum time between \nreadings [ms] (all units)") -> ()  [unwired: 1 out]
      n339 = for {
        tunnel: w635 -> [w647]
        tunnel: [w646] -> w628
        tunnel: w634 -> [w648]
        tunnel: [w645] -> w607
        tunnel: w633 -> [w653] mode=indexing
        tunnel: w619 -> [w655]
        tunnel: w632 -> [w652] mode=indexing
        tunnel: w631 -> [w651] mode=indexing
        tunnel: w630 -> [w650] mode=indexing
        i -> [w654]
        # "Iterate over all sets of data, only display the one selected"
        n340 = Equal?(x=w655, y=w654) -> (x = y?=w649:bool)
        n341 = case shown="True" w649 {
          tunnel: w653 -> [_ w663]
          tunnel: w652 -> [_ w658]
          tunnel: w651 -> [_ w662]
          tunnel: w650 -> [_ w661]
          tunnel: w648 -> [w657 w659]
          tunnel: w647 -> [w656 w660]
          tunnel: [w656 w660] -> w646
          tunnel: [w657 w659] -> w645
          frame False {
            # "Do nothing"
          }
          frame True {
            # "Display data"
            "Range Exceeded" <- w661
            "Error Present" <- w663
            "Error Text" <- w662
            "Meas. Data (for active device)" <- w658
          }
        }
      }
      n342 = local read "Z"() -> (w614:dbl[])
      n343 = Index Array(array=w617, index=w619) -> (element=w618:u8)
      n344 = Index Array(array=w621, index=w619) -> (element=w609:dbl)
      n345 = Index Array(array=w614, index=0) -> (element=w605:dbl)
      n346 = Replace Array Subset(array=w621, new element=w605, index=w619) -> (w622:dbl[])
      n347 = Index Array(array=w606, index=w619) -> (element=w620:string)
      n348 = Index Array(array=w624, index=w619) -> (element=w623:T12)
      n349 = call "Write SetPoint_no prev.vi"("Setpoint"=w605, "Previous Setpoint"=w609, "Unit ID (A)"=w620, "error in"=w628, "Software Version"=w618, "Controller Info out"=w623, "VISA Session In"=w607) -> ("error out"=w627:errorcluster, "Controller Info out"=w625:T12, "VISA Session Out"=w608:refnum<visa-resource-name>)  [unwired: 1 in, 1 out]
      n350 = Replace Array Subset(array=w624, new element=w625, index=w619) -> (w626:T13)
      n351 = call <extravilib>:"Read.vi"("channel"=w615) -> ("element"=w616:bool)  [unwired: 1 in, 1 out]
    }
    n352 = while "Hold Setpoints" {
      tunnel: w12 -> [w53]
      stop <- w54 stop-if-true
      n353 = call-poly <vilib>:"Read Delimited Spreadsheet.vi"("file path (dialog if empty)"="Read File", "start of read offset (chars.:0)"=0, "delimiter (\\t)"="," ("delimiter (\\t)")) -> ("all rows"=w49:dbl[][])  [unwired: 7 in, 5 out]
      "all rows" <- w49
      n354 = Array Subset(array=w49, index (row)="Start From:") -> (w47:dbl[][])  [unwired: 3 in]
      "Setpoints" <- w47
      n355 = Array Size(array=w47) -> (size(s)=w56:i32[])
      n356 = Index Array(array=w56, index=0) -> (element=→"len_SP":i32)
      n357 = call <extravilib>:"Read.vi"("channel"=w53) -> ("element"=w54:bool)  [unwired: 1 in, 1 out]
    }
    n358 = VISA Close(VISA resource name=w41, error in (no error)=w40) -> (error out=w42:errorcluster)
    n359 = Initialize Array(0.0 ("element"), 2 ("dimension size")) -> (→"Z":dbl[])
    n360 = call <vilib>:"Simple Error Handler.vi"("error in (no error)"=w42) -> ("error?"=w4:bool)  [unwired: 4 in, 4 out]
    n361 = call "CalibrationAlerts.vi"("Alert Type (0)"=5, "Trigger"=w4) -> ()  [unwired: 10 in]
    n362 = call-poly <vilib>:"Write Delimited Spreadsheet.vi"("file path (dialog if empty)"="Write File", "1D data"=string[] ["Date/Time", "Time [hh:mm:ss]", "Device ID", "P_MFC [psia]", "T_MFC [C]", "Volume Flow [LPM]", "Mass Flow [SLPM]", "SP_MFC [LPM]", "T_SCh [C]", "Iter_#", "V_D [V]", "V_H [V]", "Iter_Duration [ms]", "C_SP_CH4 [ppm]", "C_SP_H2S [ppm]"], "append to file? (new file:F)"=TRUE, "delimiter (\\t)"="," ("delimiter (\\t)")) -> ()  [unwired: 10 in, 2 out]
    n363 = node-c288(w45) -> ()  [unwired: 1 out]
  }
